vi "start_get_request.vi"(7 "save_to_file":path, 8 "error in (no error)":errorcluster, 9 "Headers in":refnum<class "Headers.lvclass">, 10 "url":string, 11 "Client in":refnum<class "Client.lvclass">) -> (0 "error out":errorcluster, 2 "Request":refnum<class "Request.lvclass">, 3 "Client out":refnum<class "Client.lvclass">)   [LabVIEW 2020]
uses:
  Client.lvclass
  Request/Request.lvclass
  Headers/Headers.lvclass
  Types/http_method_enum.ctl
  RequestBuilder/RequestBuilder.lvclass
  reqwest.lvlib
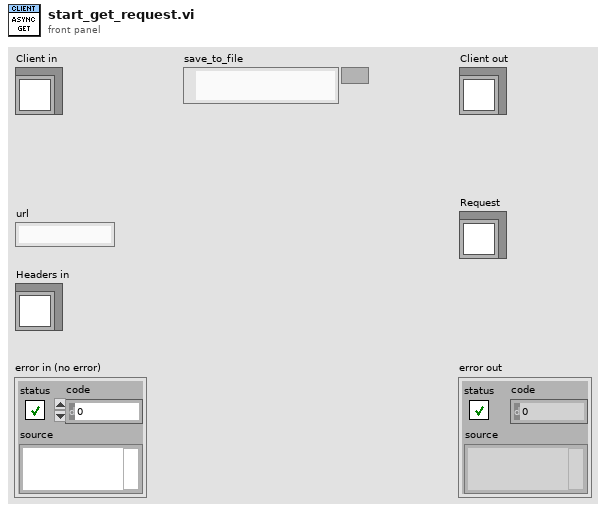
[diagram p1: front panel]
types:
  T1 = typedef "reqwest.lvlib/http_method_enum.ctl" = enum8{"<select>", "GET", "POST", "PUT", "DELETE", "HEAD", "OPTIONS", "CONNECT", "PATCH", "TRACE"}
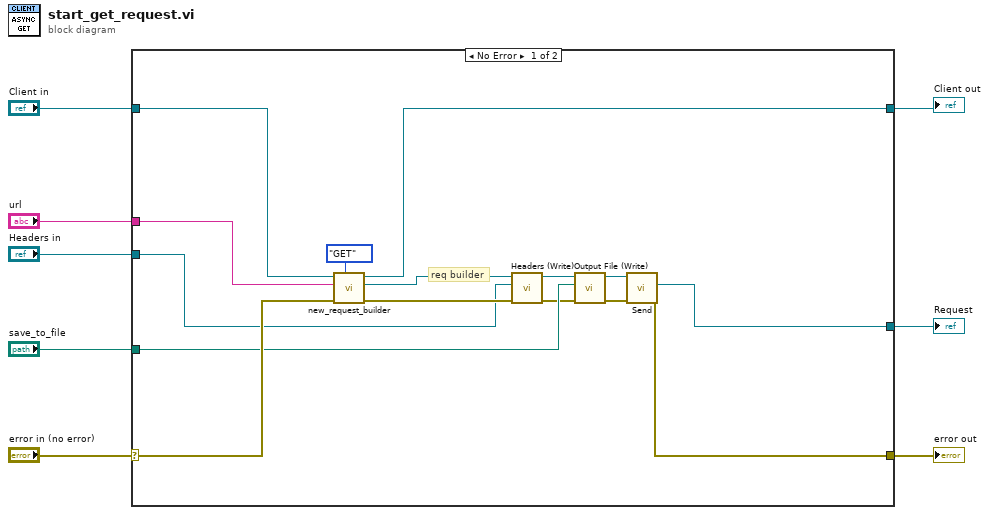
[diagram p0: block diagram]
diagram:
  n1 = case shown="No Error" "error in (no error)" {
    selector: "error in (no error)" -> [w17 w24]
    tunnel: "Client in" -> [w19 w25]
    tunnel: [w15 _] -> w6
    tunnel: [w16 w24] -> w4
    tunnel: [w20 w25] -> w5
    tunnel: "url" -> [w18 _]
    tunnel: "save_to_file" -> [w14 _]
    tunnel: "Headers in" -> [w9 _]
    frame No Error {
      # "req builder"
      n2 = call "new_request_builder.vi"("HTTP Method"=http_method_enum."GET", "error in (no error)"=w17, "url"=w18, "Client in"=w19) -> ("error out"=w11:errorcluster, "RequestBuilder out"=w13:refnum<class "RequestBuilder.lvclass">, "Client out"=w20:refnum<class "Client.lvclass">)  [unwired: 5 in]
      n3 = call "Headers (Write).vi"("error in (no error)"=w11, "Headers"=w9, "obj in"=w13) -> ("error out"=w10:errorcluster, "obj out"=w12:refnum<class "RequestBuilder.lvclass">)  [unwired: 6 in, 1 out]
      n4 = call "Output File (Write).vi"("error in (no error)"=w10, "output_file"=w14, "obj in"=w12) -> ("error out"=w22:errorcluster, "obj out"=w23:refnum<class "RequestBuilder.lvclass">)  [unwired: 6 in, 1 out]
      n5 = call "Send.vi"("error in (no error)"=w22, "obj in"=w23) -> ("error out"=w16:errorcluster, "request"=w15:refnum<class "Request.lvclass">)  [unwired: 8 in]
    }
    frame Error {
    }
  }
  "error out" <- w4
  "Request" <- w6
  "Client out" <- w5
